vi "RELEASE - 1.1 - Solenoid 1Button - David G.vi"(10 "?":bool=TRUE, 11 "refnum name":string="My Solenoid RefNum") -> ()   [LabVIEW 2019]
uses:
  <vilib>/Rock Robotics/WPI/Solenoid/WPI_SolenoidValue.ctl
  <vilib>/Rock Robotics/WPI/Solenoid/WPI_SolenoidSetEnum.vi
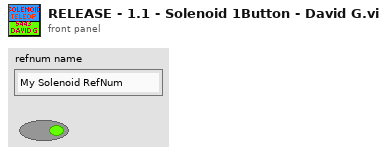
[diagram p1: front panel]
types:
  T1 = typedef "WPI_SolenoidValue.ctl" = enum16{"Off", "On", "Forward", "Reverse"}
  T2 = typedef "WPI_SolenoidDevRef.ctl" = cluster{"DevStatus":errorcluster, "Pneumatics Control Module":u8, "Forward Solenoid Channel":T3, "Reverse Solenoid Channel":T3}
  T3 = typedef "WPI_SolenoidChannel.ctl" = enum8{"Solenoid 0", "Solenoid 1", "Solenoid 2", "Solenoid 3", "Solenoid 4", "Solenoid 5", "Solenoid 6", "Solenoid 7", "Invalid"}
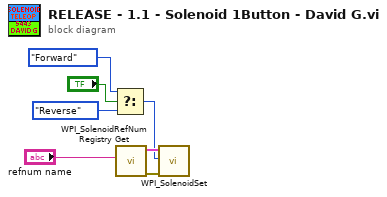
[diagram p0: block diagram]
diagram:
  n1 = Select(t=WPI_SolenoidValue."Forward" ("Value"), s="?", f=WPI_SolenoidValue."Reverse" ("Value")) -> (s? t:f=w6:T1)
  n2 = call <vilib>:"WPI_SolenoidRefNum Registry Get.vi"("refnum name"="refnum name") -> ("error out"=w3:errorcluster, "SolenoidDevRef"=w7:T2)  [unwired: 9 in]
  n3 = call-poly <vilib>:"WPI_SolenoidSet.vi"("error in (no error)"=w3, "Value"=w6, "SolenoidDevRef"=w7) -> ()  [unwired: 7 in, 2 out]
